vi "Write Data.vi"(8 "error in (no error)":errorcluster, 10 "Data":bool, 11 "Boolean Data in":refnum<class "Boolean Data.lvclass">) -> (0 "error out":errorcluster, 3 "Boolean Data out":refnum<class "Boolean Data.lvclass">)   [LabVIEW 2015, in "Boolean Data.lvclass"]
uses:
  Boolean Data.lvclass
  Boolean Data.lvclass/Boolean Data.ctl
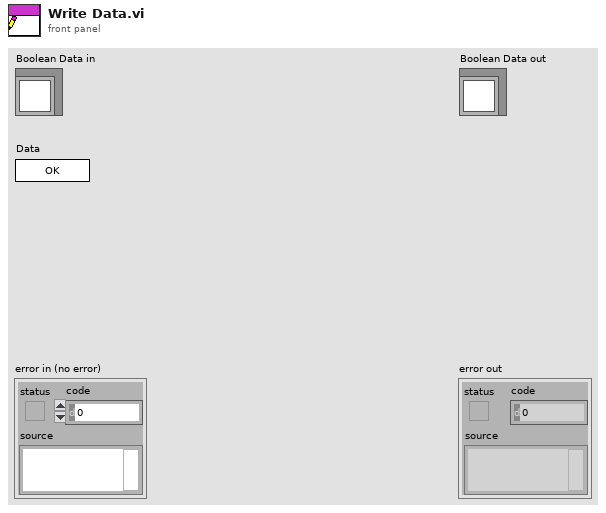
[diagram p1: front panel]
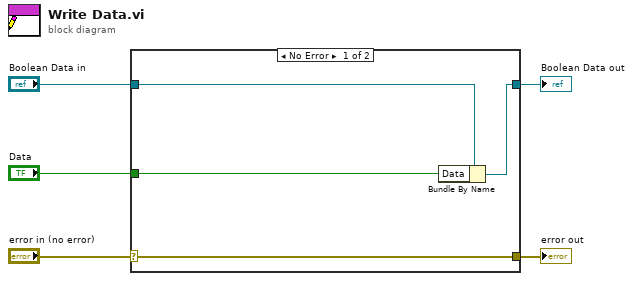
[diagram p0: block diagram]
diagram:
  n1 = case shown="No Error" "error in (no error)" {
    selector: "error in (no error)" -> [w9 w10]
    tunnel: [w9 w10] -> w4
    tunnel: [w7 w11] -> w2
    tunnel: "Boolean Data in" -> [w8 w11]
    tunnel: "Data" -> [w6 _]
    frame No Error {
      n2 = Bundle By Name(cluster=w8, "Data"=w6) -> (w7:refnum<class "Boolean Data.lvclass">)
    }
    frame Error {
    }
  }
  "error out" <- w4
  "Boolean Data out" <- w2
